vi "Filter Shortcut Menu Activation Event.vi"(8 "error in (no error)":errorcluster, 10 "ShortcutMenuActivationMsg":refnum<class "ShortcutMenuActivationMsg.lvclass">, 11 "File Explorer Event Filter in":refnum<class "File Explorer Event Filter.lvclass">) -> (0 "error out":errorcluster, 1 "Discard?":bool, 3 "File Explorer Event Filter out":refnum<class "File Explorer Event Filter.lvclass">)   [LabVIEW 2020, in "File Explorer.lvlib" / "File Explorer Event Filter.lvclass"]
doc: "Calls the overridable \"Handle Run time menu item select.vi\" that allows enables the customization of right click shortcut run time menus on the tree."
uses:
  <vilib>/gpm_packages/@cs/file-explorer-extension/Source/File Explorer/File Explorer Event Filter/File Explorer Event Filter.lvclass
  <vilib>/gpm_packages/@cs/mva-viewable/Source/ActorEvents/IEventAggregator Messages/ShortcutMenuActivationMsg/ShortcutMenuActivationMsg.lvclass
  <vilib>/gpm_packages/@cs/file-explorer-extension/Source/File Explorer/File Explorer Event Filter/File Explorer Event Filter.lvclass/File Explorer Event Filter.ctl
  <vilib>/gpm_packages/@cs/mva-viewable/Source/ActorEvents/IEventAggregator Messages/ShortcutMenuActivationMsg/ShortcutMenuActivationMsg.lvclass/ShortcutMenuActivationMsg.ctl
  <vilib>/gpm_packages/@cs/file-explorer-extension/Source/File Explorer/File Explorer Messages/Handle Activate Menu On Tree Item Msg/Handle Activate Menu On Tree Item Msg.lvclass/Handle Activate Menu On Tree Item Msg.ctl
  <vilib>/gpm_packages/@cs/actor-framework-messages/Source/RoundTripMessage/RoundTripMessage.lvclass/RoundTripMessage.ctl
  <vilib>/ActorFramework/Message Enqueuer/Message Enqueuer.lvclass/Message Enqueuer.ctl
  <vilib>/ActorFramework/Message Enqueuer/Enqueue.vi
  <vilib>/gpm_packages/@cs/file-explorer-extension/Source/File Explorer/File Explorer Messages/Handle Activate Menu On Tree Item Msg/Handle Activate Menu On Tree Item Msg.lvclass
  C:/Program Files/National Instruments/LabVIEW 2020/vi.lib/gpm_packages/@cs/actor-framework-messages/Source/RoundTripMessage/RoundTripMessage.lvclass
  <vilib>/gpm_packages/@cs/actor-framework-messages/Source/RoundTripMessage/RoundTripMessage.lvclass
  C:/Program Files/National Instruments/LabVIEW 2020/vi.lib/ActorFramework/Message/Message.lvclass
  <vilib>/ActorFramework/Message Priority Queue/Priority Enqueue.vi
panel:
  # "No additional\nEvent Data"
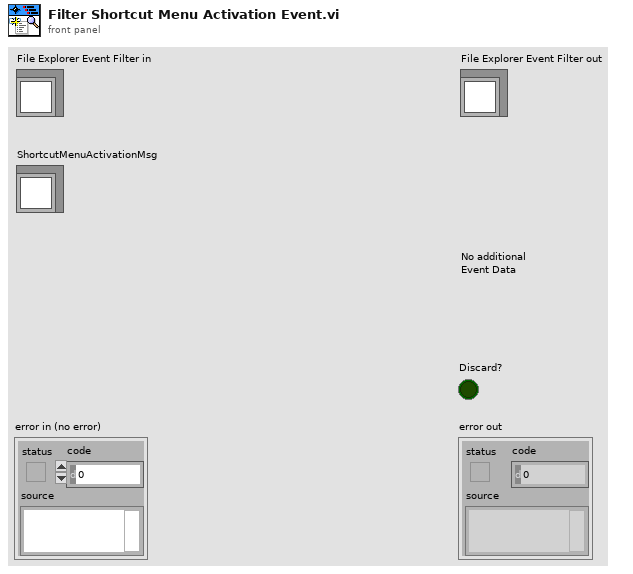
[diagram p1: front panel]
types:
  T1 = typedef "LVPoint32TypeDef.ctl" = cluster{"Horizontal":i32, "Vertical":i32}
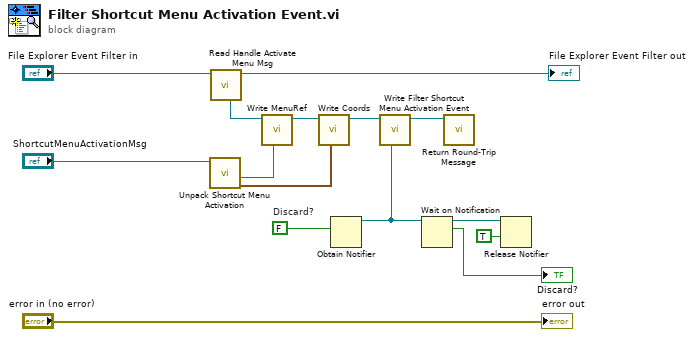
[diagram p0: block diagram]
diagram:
  w12 = FALSE  # Discard?
  n1 = call <vilib>:"Unpack Shortcut Menu Activation.vi"("ShortcutMenuActivationMsg"="ShortcutMenuActivationMsg") -> ("Coords"=w7:T1, "MenuRef"=w8:refnum<k9>)  [unwired: 5 in, 4 out]
  n2 = call <vilib>:"Read Handle Activate Menu Msg.vi"("File Explorer Event Filter in"="File Explorer Event Filter in") -> ("File Explorer Event Filter out"=→"File Explorer Event Filter out":refnum<class "File Explorer Event Filter.lvclass">, "Handle Activate Menu On Tree Item Msg"=w10:refnum<class "Handle Activate Menu On Tree Item Msg.lvclass">)  [unwired: 9 in]
  n3 = call <vilib>:"Write MenuRef.vi"("MenuRef"=w8, "Handle Activate Menu On Tree Item Msg in"=w10) -> ("Handle Activate Menu On Tree Item Msg out"=w9:refnum<class "Handle Activate Menu On Tree Item Msg.lvclass">)  [unwired: 9 in]
  n4 = call <vilib>:"Write Coords.vi"("Coordinates"=w7, "Handle Activate Menu On Tree Item Msg in"=w9) -> ("Handle Activate Menu On Tree Item Msg out"=w6:refnum<class "Handle Activate Menu On Tree Item Msg.lvclass">)  [unwired: 9 in]
  n5 = Obtain Notifier(notification data type=w12) -> (notifier out=w5:refnum<notifier>)  [unwired: 3 in, 2 out]
  n6 = call <vilib>:"Write Filter Shortcut Menu Activation Event.vi"("Filter Shortcut Menu Activation Event"=w5, "Handle Activate Menu On Tree Item Msg in"=w6) -> ("Handle Activate Menu On Tree Item Msg out"=w1:refnum<class "Handle Activate Menu On Tree Item Msg.lvclass">)  [unwired: 9 in]
  n7 = Wait on Notification(notifier=w5) -> (notifier out=w4:refnum<notifier>, notification=→"Discard?":bool)  [unwired: 3 in, 2 out]
  n8 = call <vilib>:"Return Round-Trip Message.vi"("RoundTripMessage In"=w1) -> ()  [unwired: 10 in, 1 out]
  n9 = Release Notifier(notifier=w4, force destroy? (F)=TRUE) -> ()  [unwired: 1 in, 3 out]
  "error out" <- "error in (no error)"
